vi "Read Decimal.vi"(11 "MsgSerializer":refnum<class "MsgSerializer.JSON.lvclass">) -> (2 "Decimal":T1, 3 "MsgSerializer":refnum<class "MsgSerializer.JSON.lvclass">)   [LabVIEW 2013]
uses:
  decimal-notation -- enum.ctl
  MsgSerializer/MsgSerializer.JSON.lvclass
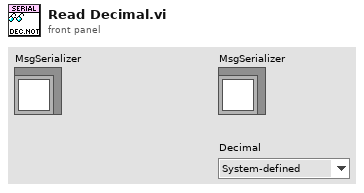
[diagram p1: front panel]
types:
  T1 = typedef "Caraya.lvlib/MsgSerializer.JSON.lvclass/decimal-notation -- enum.ctl" = enum16{"System-defined", "dot-notation", "comma-notation"}
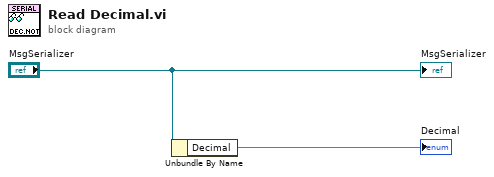
[diagram p0: block diagram]
diagram:
  n1 = Unbundle By Name("MsgSerializer") -> ("Decimal"=→"Decimal")
  "MsgSerializer" <- "MsgSerializer"
